vi "Node - Write U8 Array into Byte Buffer.vi"(8 "error in (no error)":errorcluster, 10 "U8 Array In":u8[][](array[numeric]), 11 "Node Data In":T1) -> (0 "error out":errorcluster, 3 "Node Data Out":T1)   [LabVIEW 2016, in "PXImc Router.lvlib"]
uses:
  PXImc Router.lvlib
  Controls/Node Data.ctl
  <vilib>/NI Veristand/VeriStand Data/Byte Buffer/Byte Buffer.lvclass
  Controls/Node/Node - PXImc Parameters.ctl
  Controls/Node/Transfer Data.ctl
  Controls/Node/Node Ch Properties.ctl
  Controls/Data Type.ctl
  <vilib>/NI Veristand/VeriStand Data/Byte Buffer/Byte Buffer.lvclass/Byte Buffer.ctl
  <vilib>/NI Veristand/VeriStand Data/Pointer Operations/Pointer.Write (1D U8).vi
  <vilib>/NI Veristand/VeriStand Data/VeriStand Data.lvlib
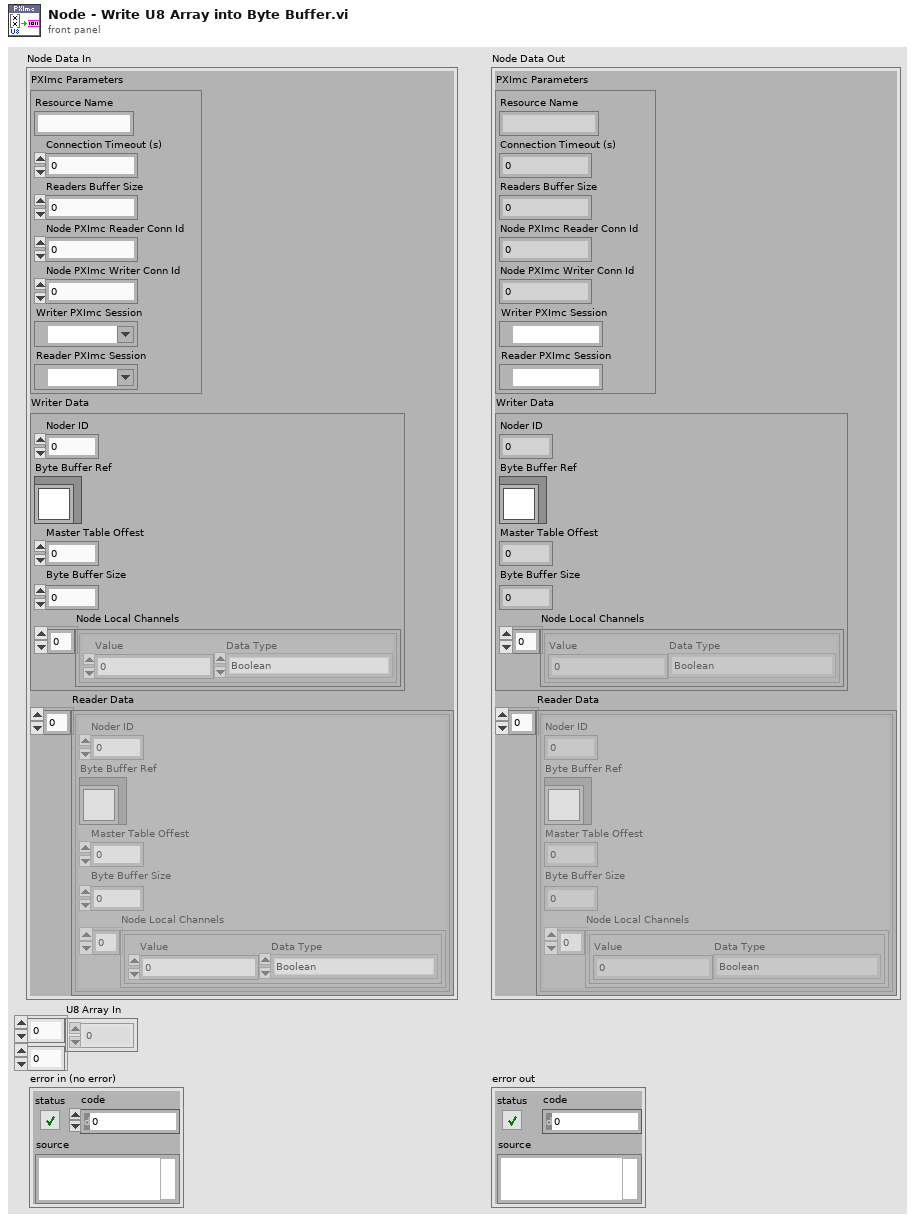
[diagram p1: front panel]
types:
  T1 = typedef "PXImc Router.lvlib/Node Data.ctl" = cluster{"PXImc Parameters":T2, "Writer Data":T3, "Reader Data":T3[]}
  T2 = typedef "PXImc Router.lvlib/Node - PXImc Parameters.ctl" = cluster{"Resource Name":string, "Connection Timeout (s)":dbl, "Readers Buffer Size":u32, "Node PXImc Reader Conn Id":u16, "Node PXImc Writer Conn Id":u16, "Writer PXImc Session":refnum<k21>, "Reader PXImc Session":refnum<k21>}
  T3 = typedef "PXImc Router.lvlib/Transfer Data.ctl" = cluster{"Noder ID":u32, "Byte Buffer Ref":refnum<class "Byte Buffer.lvclass">, "Master Table Offest":u32, "Byte Buffer Size":u32, "Node Local Channels":T4[]}
  T4 = typedef "PXImc Router.lvlib/Node Ch Properties.ctl" = cluster{"Value":dbl, "Data Type":T5}
  T5 = typedef "PXImc Router.lvlib/Data Type.ctl" = enum16{"Boolean", "SGL", "DBL", "I8", "I16", "I32", "I64", "U8", "U16", "U32", "U64"}
  T6 = typedef "VeriStand Data.lvlib/Byte Buffer.lvclass/Byte Buffer.Pointers.ctl" = cluster{"buffer data ptr":u64, "buffer size ptr":u64, "byte order ptr":u64}
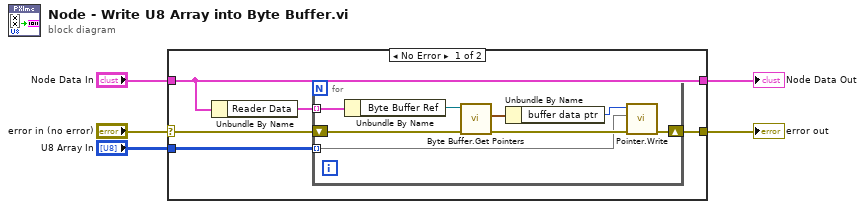
[diagram p0: block diagram]
diagram:
  n1 = case shown="No Error" "error in (no error)" {
    selector: "error in (no error)" -> [w9 w19]
    tunnel: [w8 w19] -> w2
    tunnel: "Node Data In" -> [w10 w20]
    tunnel: [w10 w20] -> w3
    tunnel: "U8 Array In" -> [w6 _]
    frame No Error {
      n2 = Unbundle By Name(w10) -> ("Reader Data"=w7:T3[])
      n3 = for {
        shift-right: [w14] -> w8
        shift-left: w9 -> [w17]
        tunnel: w7 -> [w13] mode=indexing
        tunnel: w6 -> [w11] mode=indexing
        n4 = Unbundle By Name(w13) -> ("Byte Buffer Ref"=w12:refnum<class "Byte Buffer.lvclass">)
        n5 = call <vilib>:"Byte Buffer.Get Pointers.vi"("error in (no error)"=w17, "Byte Buffer in"=w12) -> ("error out"=w15:errorcluster, "Byte Buffer pointers"=w18:T6)  [unwired: 7 in, 1 out]
        n6 = Unbundle By Name(w18) -> ("buffer data ptr"=w16:u64)
        n7 = call-poly <vilib>:"Pointer.Write.vi"("error in (no error)"=w15, "values"=w11, "pointer in"=w16) -> ("error out"=w14:errorcluster)  [unwired: 6 in, 2 out]
      }
    }
    frame Error {
    }
  }
  "error out" <- w2
  "Node Data Out" <- w3
